vi "Read Pressure.vi"(8 "error in (no error)":errorcluster, 11 "Model in":refnum<class "Model.lvclass">) -> (0 "error out":errorcluster, 3 "Model out":refnum<class "Model.lvclass">)   [LabVIEW 2015, in "Model.lvclass"]
uses:
  Model.lvclass
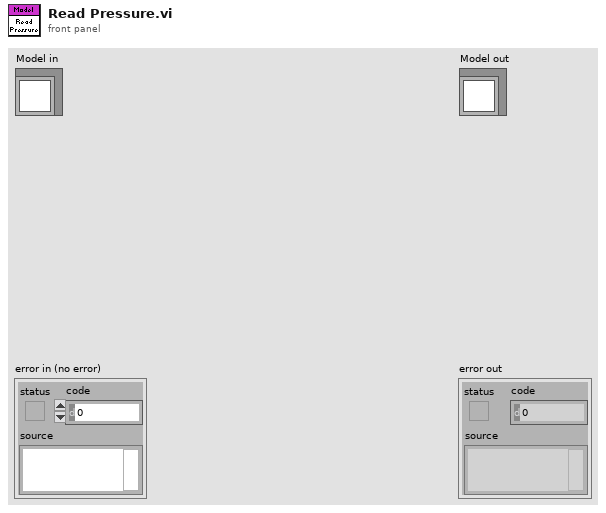
[diagram p1: front panel]
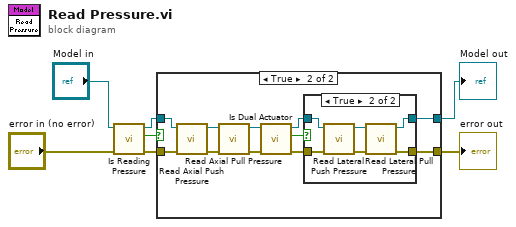
[diagram p0: block diagram]
diagram:
  n1 = call "Is Reading Pressure.vi"("error in (no error)"="error in (no error)", "Model in"="Model in") -> ("error out"=w4:errorcluster, "Is Reading Pressure"=w5:bool, "Model out"=w3:refnum<class "Model.lvclass">)  [unwired: 7 in]
  n2 = case shown="True" w5 {
    tunnel: [w8 w19] -> w7
    tunnel: [w9 w17] -> w6
    tunnel: w4 -> [w8 w16]
    tunnel: w3 -> [w9 w15]
    frame False {
    }
    frame True {
      n3 = call "Read Axial Push Pressure.vi"("error in (no error)"=w16, "Model in"=w15) -> ("error out"=w20:errorcluster, "Model out"=w18:refnum<class "Model.lvclass">)  [unwired: 8 in]
      n4 = call "Read Axial Pull Pressure.vi"("error in (no error)"=w20, "Model in"=w18) -> ("error out"=w10:errorcluster, "Model out"=w11:refnum<class "Model.lvclass">)  [unwired: 8 in]
      n5 = call "Is Dual Actuator.vi"("error in (no error)"=w10, "Model in"=w11) -> ("error out"=w13:errorcluster, "Is Dual Actuator"=w14:bool, "Model out"=w12:refnum<class "Model.lvclass">)  [unwired: 7 in]
      n6 = case shown="True" w14 {
        tunnel: [w21 w27] -> w19
        tunnel: [w22 w25] -> w17
        tunnel: w13 -> [w21 w24]
        tunnel: w12 -> [w22 w23]
        frame False {
        }
        frame True {
          n7 = call "Read Lateral Push Pressure.vi"("error in (no error)"=w24, "Model in"=w23) -> ("error out"=w28:errorcluster, "Model out"=w26:refnum<class "Model.lvclass">)  [unwired: 8 in]
          n8 = call "Read Lateral Pull Pressure.vi"("error in (no error)"=w28, "Model in"=w26) -> ("error out"=w27:errorcluster, "Model out"=w25:refnum<class "Model.lvclass">)  [unwired: 8 in]
        }
      }
    }
  }
  "error out" <- w7
  "Model out" <- w6
